vi "UTIL_FillorDrain.vi"(11 "PVs":dbl) -> (3 "Boolean":bool)   [LabVIEW 2024]
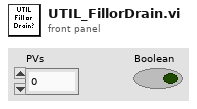
[diagram p1: front panel]
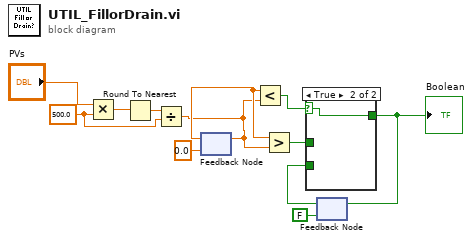
[diagram p0: block diagram]
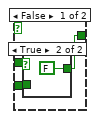
[diagram p2: hidden frame]
diagram:
  w2 = 500.0 ("y")
  n1 = Multiply(x="PVs", y=w2) -> (x*y=w4:dbl)
  n2 = Round To Nearest(number=w4) -> (nearest integer value=w3:dbl)
  n3 = Divide(x=w3, y=w2) -> (x/y=w1:dbl)
  n4 = feedback #1(0.0 ("PVs")) -> (w7:dbl)
  n5 = feedback-in #1(w1) -> ()
  n6 = Less?(x=w7, y=w1) -> (x < y?=w8:bool)
  n7 = Greater?(x=w7, y=w1) -> (0:w9:bool)
  n8 = feedback #2(FALSE) -> (w11:bool)
  n9 = case shown="True" w8 {
    selector: w8 -> [_ w18]
    tunnel: [w14 w18] -> w10
    tunnel: w9 -> [w15 _]
    tunnel: w11 -> [w13 _]
    frame False {
      n10 = case shown="True" w15 {
        tunnel: [w16 FALSE] -> w14
        tunnel: w13 -> [w16 _]
        frame False {
        }
        frame True {
        }
      }
    }
    frame True {
    }
  }
  "Boolean" <- w10
  n11 = feedback-in #2(w10) -> ()
